vi "Launch Configurable Nested Actor.vi"(6 "Open Actor Core front panel? (F)":bool, 7 "Configuration":variant, 8 "error in (no error)":errorcluster, 9 "Name":string, 10 "Configurable Dependency":refnum<class "ConfigurableActor.lvclass">, 11 "Actor":refnum<class "Actor.lvclass">) -> (0 "error out":errorcluster)   [LabVIEW 2014, in "ConfigurableActor.lvclass"]
uses:
  ConfigurableActor.lvclass
  <vilib>/ActorFramework/Actor/Actor.lvclass
  <vilib>/ActorFramework/Actor/Actor.lvclass/Actor.ctl
  <vilib>/ActorFramework/Message Enqueuer/Message Enqueuer.lvclass/Message Enqueuer.ctl
  ConfigurableActor.lvclass/ConfigurableActor.ctl
  <vilib>/LabVIEW Open Source Project/Unicity/UniqueName/UniqueNameClass/UniqueName.lvclass/UniqueName.ctl
  <vilib>/ActorFramework/Message Enqueuer/Init from Existing Queue.vi
  <vilib>/ActorFramework/Message Enqueuer/Message Enqueuer.lvclass
  <vilib>/LabVIEW Open Source/Configuration Manager/Manager/ConfigManager.lvclass
  <vilib>/LabVIEW Open Source Project/Unicity/UniqueName/Registry/NameRegistry.lvclass
  <vilib>/LabVIEW Open Source Project/Unicity/UniqueName/UniqueNameClass/UniqueName.lvclass
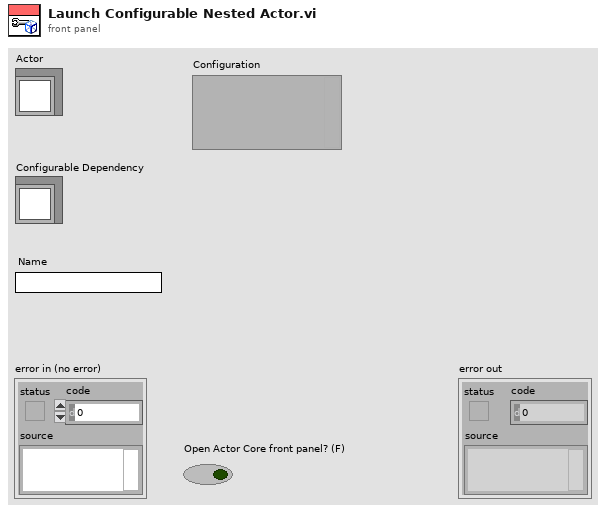
[diagram p1: front panel]
types:
  T1 = typedef "UniqueName.lvlib/NameRegistry.lvclass/RegistryConfiguration.ctl" = cluster{"Delimiter":refnum<class "Delimiter.lvclass">, "RandomStringGenerator":refnum<class "RandomStringGenerator.lvclass">, "UniquenessCriteria":refnum<class "UniquenessCriteria.lvclass">, "StringIncrement":refnum<class "StringIncrement.lvclass">}
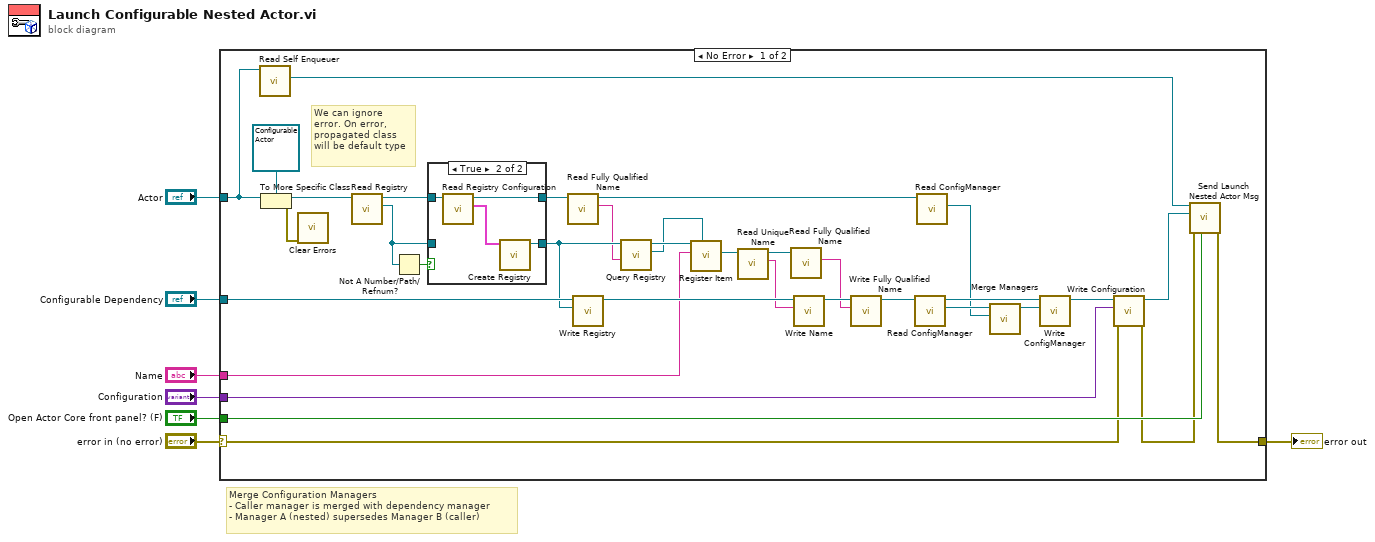
[diagram p0: block diagram]
diagram:
  # "Merge Configuration Managers\n- Caller manager is merged with dependency manager\n- Manager A (nested) supersedes Manager B (caller)"
  n1 = case shown="No Error" "error in (no error)" {
    selector: "error in (no error)" -> [w29 w48]
    tunnel: [w37 w48] -> w6
    tunnel: "Actor" -> [w27 _]
    tunnel: "Configurable Dependency" -> [w20 _]
    tunnel: "Open Actor Core front panel? (F)" -> [w38 _]
    tunnel: "Name" -> [w13 _]
    tunnel: "Configuration" -> [w30 _]
    frame No Error {
      # "We can ignore\nerror. On error,\npropagated class\nwill be default type"
      n2 = call <vilib>:"Read Self Enqueuer.vi"("Actor"=w27) -> ("Self Enqueuer"=w26:refnum<class "Message Enqueuer.lvclass">)  [unwired: 10 in]
      n3 = To More Specific Class(target class=refnum<class "ConfigurableActor.lvclass"> refnum ("ConfigurableActor.lvclass"), reference=w27) -> (specific class reference=w24:refnum<class "ConfigurableActor.lvclass">, error out=w22:errorcluster)  [unwired: 1 in]
      n4 = call <vilib>:"Clear Errors.vi"("error in (no error)"=w22) -> ()  [unwired: 5 in, 2 out]
      n5 = call "Read Registry.vi"("ConfigurableActor in"=w24) -> ("Registry"=w21:refnum<data-value>, "ConfigurableActor out"=w9:refnum<class "ConfigurableActor.lvclass">)  [unwired: 9 in]
      n6 = Not A Number/Path/Refnum?(number/path/refnum=w21) -> (NaN/Path/Refnum?=w23:bool)
      n7 = case shown="True" w23 {
        tunnel: [w43 w47] -> w18
        tunnel: w21 -> [w43 _]
        tunnel: w9 -> [w42 w46]
        tunnel: [w42 w45] -> w8
        frame False {
        }
        frame True {
          n8 = call "Read Registry Configuration.vi"("ConfigurableActor in"=w46) -> ("Registry Configuration"=w44:T1, "ConfigurableActor out"=w45:refnum<class "ConfigurableActor.lvclass">)  [unwired: 9 in]
          n9 = call <vilib>:"Create Registry.vi"("Registry Configuration"=w44) -> ("Registry"=w47:refnum<data-value>)  [unwired: 9 in, 1 out]
        }
      }
      n10 = call <vilib>:"Read Fully Qualified Name.vi"("ConfigurableActor in"=w8) -> ("Fully Qualified Name"=w17:string, "ConfigurableActor out"=w25:refnum<class "ConfigurableActor.lvclass">)  [unwired: 8 in, 1 out]
      n11 = call "Write Registry.vi"("Registry"=w18, "ConfigurableActor in"=w20) -> ("ConfigurableActor out"=w19:refnum<class "ConfigurableActor.lvclass">)  [unwired: 9 in]
      n12 = call <vilib>:"Query Registry.vi"("Search string"=w17, "Registry in"=w18) -> ("Node"=w15:refnum<class "UniqueName.lvclass">, "Registry"=w16:refnum<data-value>)  [unwired: 5 in, 3 out]
      n13 = call <vilib>:"Register Item.vi"("Owner"=w15, "New Object Name"=w13, "Registry in"=w16) -> ("New Node"=w14:refnum<class "UniqueName.lvclass">)  [unwired: 6 in, 2 out]
      n14 = call <vilib>:"Read Unique Name.vi"("UniqueName in"=w14) -> ("Unique Name"=w12:string, "UniqueName out"=w11:refnum<class "UniqueName.lvclass">)  [unwired: 9 in]
      n15 = call <vilib>:"Read Fully Qualified Name.vi"("UniqueName in"=w11) -> ("Fully Qualified Name"=w10:string)  [unwired: 9 in, 1 out]
      n16 = call "Write Name.vi"("Name"=w12, "ConfigurableActor in"=w19) -> ("ConfigurableActor out"=w34:refnum<class "ConfigurableActor.lvclass">)  [unwired: 8 in, 1 out]
      n17 = call "Write Fully Qualified Name.vi"("Fully Qualified Name"=w10, "ConfigurableActor in"=w34) -> ("ConfigurableActor out"=w33:refnum<class "ConfigurableActor.lvclass">)  [unwired: 8 in, 1 out]
      n18 = call "Read ConfigManager.vi"("ConfigurableActor in"=w33) -> ("ConfigManager"=w39:refnum<class "ConfigManager.lvclass">, "ConfigurableActor out"=w41:refnum<class "ConfigurableActor.lvclass">)  [unwired: 8 in, 1 out]
      n19 = call "Read ConfigManager.vi"("ConfigurableActor in"=w25) -> ("ConfigManager"=w35:refnum<class "ConfigManager.lvclass">)  [unwired: 8 in, 2 out]
      n20 = call <vilib>:"Merge Managers.vi"("ConfigManager B"=w35, "ConfigManager A"=w39) -> ("ConfigManagerCollection"=w40:refnum<class "ConfigManagerCollection.lvclass">)  [unwired: 9 in]
      n21 = call "Write ConfigManager.vi"("ConfigManager"=w40, "ConfigurableActor in"=w41) -> ("ConfigurableActor out"=w32:refnum<class "ConfigurableActor.lvclass">)  [unwired: 8 in, 1 out]
      n22 = call "Write Configuration.vi"("error in (no error)"=w29, "Type"=w30, "ConfigurableActor in"=w32) -> ("error out"=w28:errorcluster, "ConfigurableActor out"=w31:refnum<class "ConfigurableActor.lvclass">)  [unwired: 7 in]
      n23 = call <vilib>:"Send Launch Nested Actor Msg.vi"("Open Actor Core front panel? (F)"=w38, "error in"=w28, "Nested Actor"=w31, "Self Enqueuer in"=w26) -> ("error out"=w37:errorcluster)  [unwired: 6 in, 1 out]
    }
    frame Error {
    }
  }
  "error out" <- w6
